vi "Complex Compact Cholesky Factor.vi"(0 "Compact Array":cluster{"Compact Array":cdb[], "array type":i32} {"array type" items=["lower triangular", "upper triangular", "symmetric matrix"]; "Compact Array" format="%.2f"}) -> (1 "Compact Cholesky Array":cluster{"Compact Array":cdb[], "array type":i32} {"array type" items=["lower triangular", "upper triangular", "symmetric matrix"]; "Compact Array" format="%.2f"}, 2 "error":i32)   [LabVIEW 2020, in "NI_AALBase.lvlib"]
doc: "Perform Cholesky Factorization for a complex, positive definite matrix in compact storage. The output <B>Compact Cholesky Array</B> contains the factored, lower triangular matrix L in compact storage."
uses:
  <vilib>/Analysis/NI_AALBase.lvlib
  <resource>/lvanlys.dll
panel:
  # "Complex Compact Cholesky Factorization"
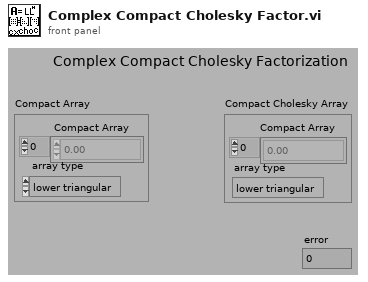
[diagram p1: front panel]
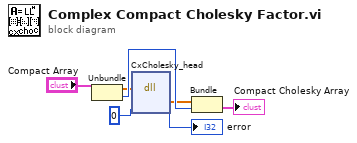
[diagram p0: block diagram]
diagram:
  n1 = Unbundle("Compact Array") -> ("Compact Array"=w5:cdb[], "array type"=w6:i32)
  n2 = dll-call lib="e:/builds/penguin/labview/branches/2020/dev/dist/resource/lvanlys.*" fn="CxCholesky_head"("Compact Array"=w5, 0) -> ("Compact Array"=w4:cdb[], →"error":i32)  [unwired: 4 in, 2 out]
  n3 = Bundle("Compact Array"=w4, "array type"=w6) -> (→"Compact Cholesky Array":cluster{"Compact Array":cdb[], "array type":i32})  [unwired: 1 in]
